vi "Disabled.vi"(7 "Robot Mode":T2, 10 "Match Info":T1={"Autonomous Elapsed Seconds"=0.0, "TeleOp Elapsed Seconds"=0.0, "Disabled Elapsed Seconds"=0.0, "Visited Autonomous"=FALSE, "Visited TeleOp"=FALSE, "Visited Disabled"=FALSE, "Autonomous Settings"={"Autonomous Style"=enum."Independent", "VI Refnum"=refnum}}, 11 "Call Context":T3) -> ()   [LabVIEW 2011]
doc: "This VI is called each time a disabled packet is received from the DS. It is often used to prepare for the next robot mode, to calibrate sensors, etc."
uses:
  <vilib>/Rock Robotics/WPI/DriverStation/WPI_DriverStationDerivedRobotMode.ctl
  <vilib>/Rock Robotics/WPI/DriverStation/WPI_DriverStationRobotMode.ctl
  <vilib>/Rock Robotics/WPI/DriverStation/WPI_DriverStationMatch Info.ctl
  Robot Global Data.vi
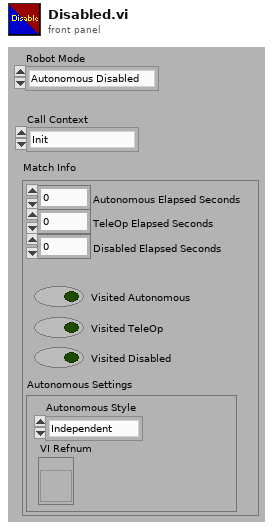
[diagram p1: front panel]
types:
  T1 = typedef "WPI_DriverStationMatch Info.ctl" = cluster{"Autonomous Elapsed Seconds":dbl, "TeleOp Elapsed Seconds":dbl, "Disabled Elapsed Seconds":dbl, "Visited Autonomous":bool, "Visited TeleOp":bool, "Visited Disabled":bool, "Autonomous Settings":cluster{"Autonomous Style":enum16{"Iterative", "Independent"}, "VI Refnum":refnum<vi>}}
  T2 = typedef "WPI_DriverStationRobotMode.ctl" = enum16{"Autonomous Disabled", "Autonomous Enabled", "Teleop Disabled", "Teleop Enabled", "Timeout", "Finish"}
  T3 = typedef "WPI_DriverStationDerivedRobotMode.ctl" = enum16{"Init", "Execute", "Stop"}
  T4 = typedef "WPI_JoystickDevRef.ctl" = cluster{"Device":T5}
  T5 = typedef "WPI_JoystickDeviceEnum.ctl" = enum16{"USB 1", "USB 2", "USB 3", "USB 4", "Kinect 1", "Kinect 2"}
  T6 = typedef "WPI_JoystickButtonState.ctl" = cluster{"Button 1":bool, "Button 2":bool, "Button 3":bool, "Button 4":bool, "Button 5":bool, "Button 6":bool, "Button 7":bool, "Button 8":bool, "Button 9":bool, "Button 10":bool, "Button 11":bool, "Button 12":bool}
  T7 = cluster{"axis 1 (x)":dbl, "axis 2 (y)":dbl, "axis 3 (throttle)":dbl, "axis 4":dbl, "axis 5":dbl, "axis 6":dbl}
  T8 = cluster{"VariableValueOut":dbl, "VariableValueOut":dbl}
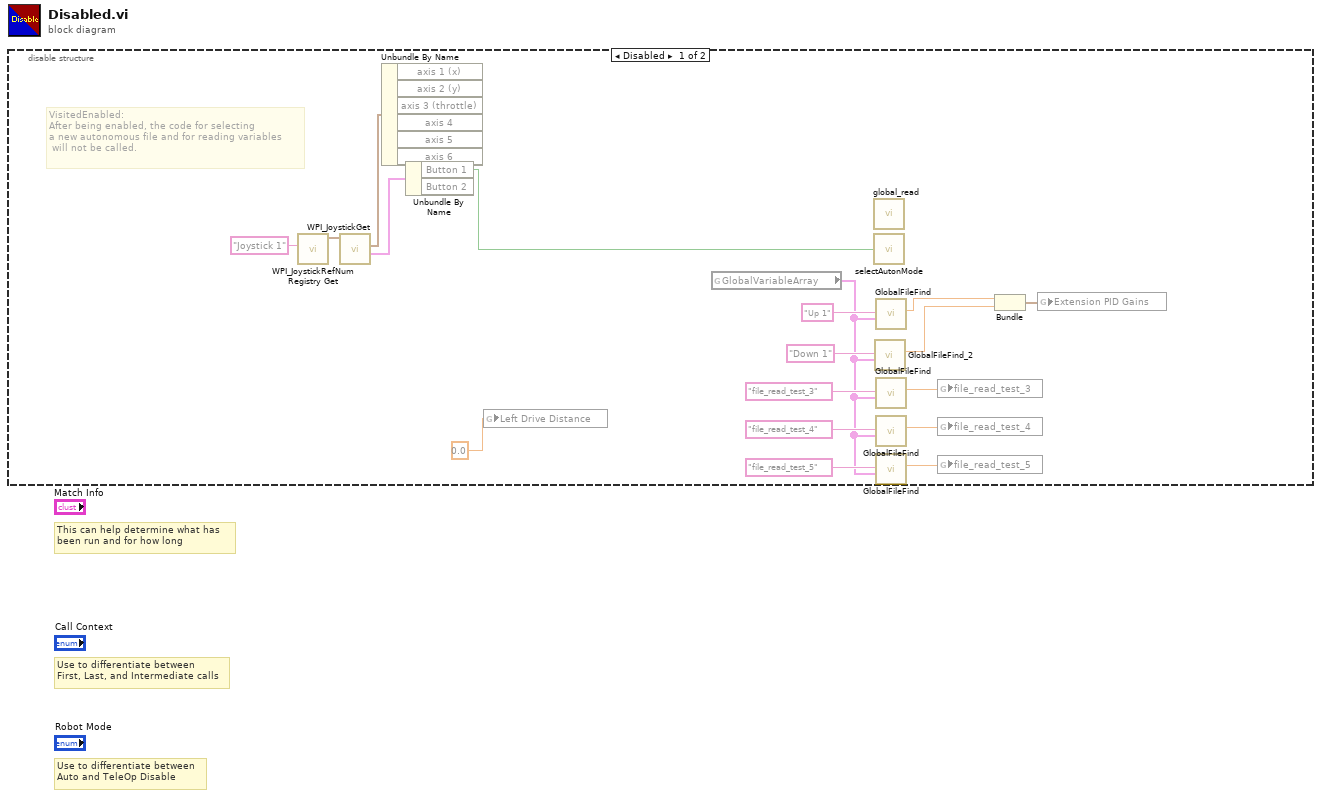
[diagram p0: block diagram]
diagram:
  # "Use to differentiate between\nFirst, Last, and Intermediate calls"
  # "This can help determine what has\nbeen run and for how long"
  # "Use to differentiate between\nAuto and TeleOp Disable"
  n1 = disable-structure shown="Disabled" {
    frame Disabled {
      # "VisitedEnabled:\nAfter being enabled, the code for selecting\na new autonomous file and for reading variables\n will not be called."
      n2 = call <vilib>:"WPI_JoystickRefNum Registry Get.vi"("refnum name"="Joystick 1") -> ("JoystickDevRef"=w17:T4)  [unwired: 1 in, 9 out]
      n3 = call <vilib>:"WPI_JoystickGet.vi"("JoystickDevRef"=w17) -> ("Buttons"=w15:T6, "Axes"=w16:T7)  [unwired: 1 in, 4 out]
      n4 = Unbundle By Name(w16) -> ()  [unwired: 6 out]
      n5 = Unbundle By Name(w15) -> ("Button 1"=w1:bool)  [unwired: 1 out]
      n6 = global write "Robot Global Data.vi" "Left Drive Distance"(0.0 ("AI 5 Setpoint")) -> ()
      n7 = global read "Robot Global Data.vi" "GlobalVariableArray"() -> (w3:cluster{"name":string, "va;":dbl}[])
      n8 = call "global_read.vi"() -> ()  [unwired: 2 in, 10 out]
      n9 = call "selectAutonMode.vi"("Joystick"=w1) -> ()  [unwired: 1 out]
      n10 = call "GlobalFileFind_2.vi"("GlobalVariableArray 2"=w3, "VariableNameLookup"="Down 1" ("refnum name")) -> ("VariableValueOut"=w2:dbl)  [unwired: 9 out]
      n11 = call "GlobalFileFind.vi"("GlobalVariableArray 2"=w3, "VariableNameLookup"="Up 1" ("refnum name")) -> ("VariableValueOut"=w6:dbl)  [unwired: 1 in, 8 out]
      n12 = call "GlobalFileFind.vi"("GlobalVariableArray 2"=w3, "VariableNameLookup"="file_read_test_3" ("refnum name")) -> ("VariableValueOut"=w9:dbl)  [unwired: 1 in, 8 out]
      n13 = call "GlobalFileFind.vi"("GlobalVariableArray 2"=w3, "VariableNameLookup"="file_read_test_4" ("refnum name")) -> ("VariableValueOut"=w13:dbl)  [unwired: 1 in, 8 out]
      n14 = call "GlobalFileFind.vi"("GlobalVariableArray 2"=w3, "VariableNameLookup"="file_read_test_5" ("refnum name")) -> ("VariableValueOut"=w10:dbl)  [unwired: 1 in, 8 out]
      n15 = global write "Robot Global Data.vi" "file_read_test_3"(w9) -> ()
      n16 = global write "Robot Global Data.vi" "file_read_test_4"(w13) -> ()
      n17 = global write "Robot Global Data.vi" "file_read_test_5"(w10) -> ()
      n18 = Bundle("VariableValueOut"=w6, "VariableValueOut"=w2) -> (w5:T8)  [unwired: 1 out]
      n19 = global write "Robot Global Data.vi" "Extension PID Gains"(w5) -> ()
    }
    frame Enabled {
    }
  }
